vi "Generate volume table.vi"(8 "error in (no error)":errorcluster, 11 "Tomo in":refnum<class "Tomo.lvclass">) -> (0 "error out":errorcluster, 2 "Volume table":dbl[][](array[numeric]), 3 "Tomo out":refnum<class "Tomo.lvclass">)   [LabVIEW 2012, in "Tomo.lvclass"]
uses:
  Tomo.lvclass
  Tomo.lvclass/Tomo.ctl
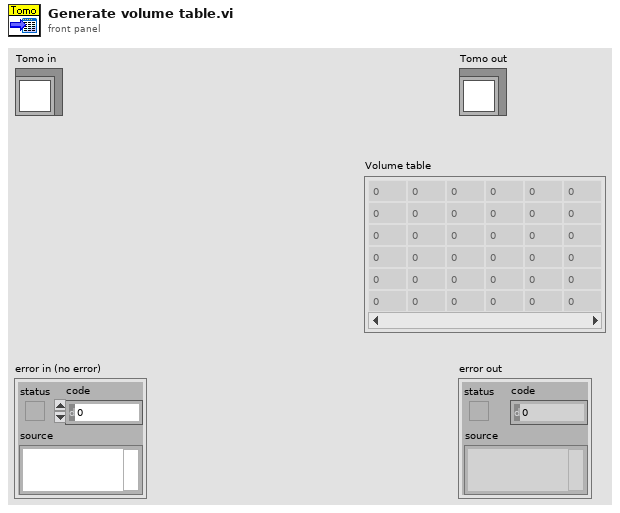
[diagram p1: front panel]
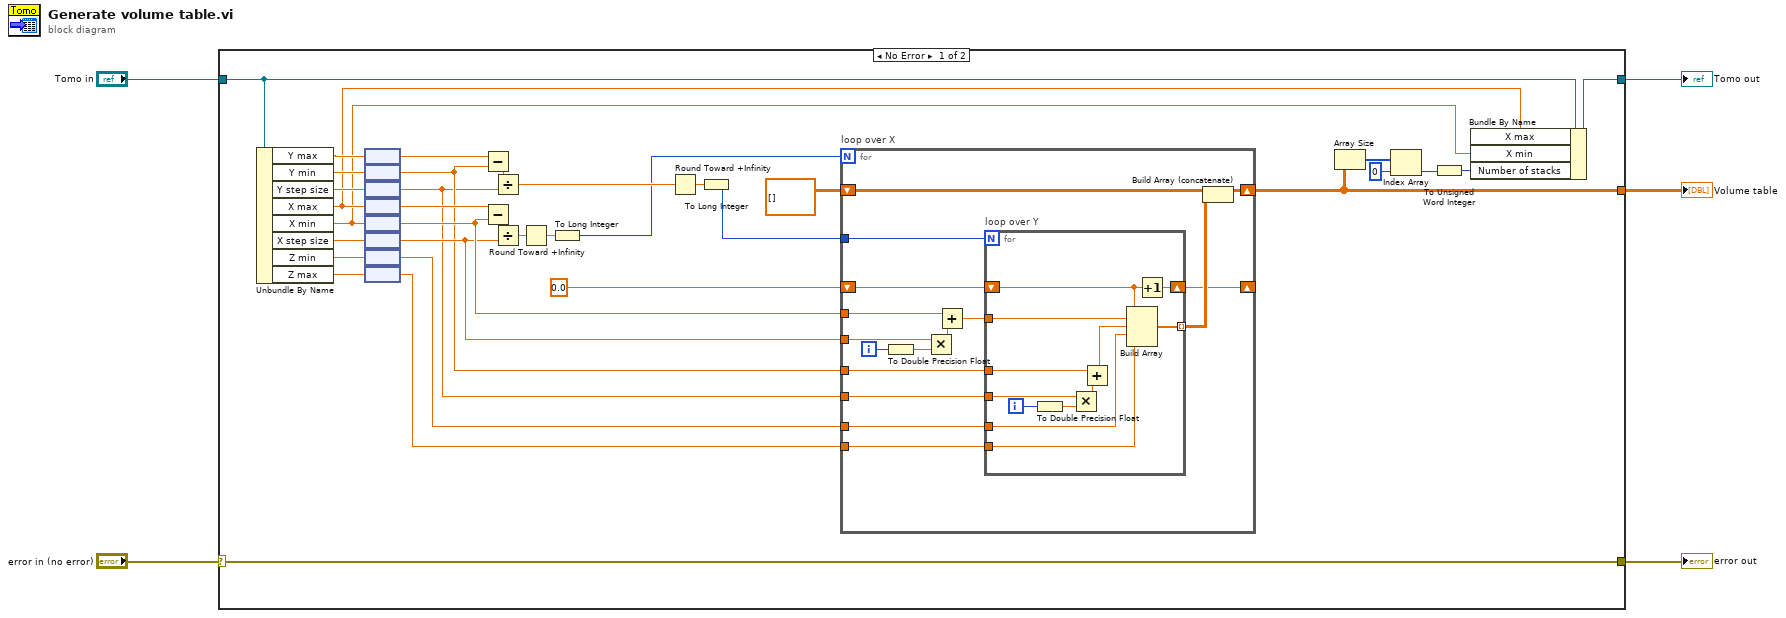
[diagram p0: block diagram]
diagram:
  n1 = case shown="No Error" "error in (no error)" {
    selector: "error in (no error)" -> [w39 w69]
    tunnel: [w39 w69] -> w4
    tunnel: [w12 w68] -> w2
    tunnel: "Tomo in" -> [w13 w68]
    tunnel: [w16 _] -> w1
    frame No Error {
      n2 = Unbundle By Name(w13) -> ("Y max"=w38:dbl[unit], "Y min"=w37:dbl[unit], "Y step size"=w36:dbl[unit], "X max"=w7:dbl[unit], "X min"=w6:dbl[unit], "X step size"=w27:dbl[unit], "Z min"=w21:dbl[unit], "Z max"=w19:dbl[unit])
      n3 = node(w38) -> (w28:dbl)
      n4 = node(w37) -> (w23:dbl)
      n5 = node(w36) -> (w22:dbl)
      n6 = node(w7) -> (w26:dbl)
      n7 = node(w6) -> (w25:dbl)
      n8 = node(w27) -> (w24:dbl)
      n9 = node(w21) -> (w20:dbl)
      n10 = node(w19) -> (w18:dbl)
      n11 = Subtract(x=w28, y=w23) -> (x-y=w35:dbl)
      n12 = Subtract(x=w26, y=w25) -> (x-y=w34:dbl)
      n13 = Divide(x=w35, y=w22) -> (x/y=w33:dbl)
      n14 = Divide(x=w34, y=w24) -> (x/y=w32:dbl)
      n15 = Round Toward +Infinity(x=w32) -> (ceil(x): smallest int >= x=w30:dbl)
      n16 = To Long Integer(number=w30) -> (32bit integer=w9:i32)
      n17 = Round Toward +Infinity(x=w33) -> (ceil(x): smallest int >= x=w31:dbl)
      n18 = To Long Integer(number=w31) -> (32bit integer=w8:i32)
      n19 = for "loop over X" {
        N: w9 -> [_]
        tunnel: w8 -> [w55]
        shift-right: [w40] -> _
        shift-left: 0.0 -> [w53]
        tunnel: w25 -> [w49]
        tunnel: w24 -> [w48]
        tunnel: w23 -> [w47]
        tunnel: w22 -> [w46]
        tunnel: w20 -> [w45]
        tunnel: w18 -> [w44]
        shift-right: [w43] -> w16
        shift-left: dbl[][] [] -> [w41]
        i -> [w54]
        n20 = To Double Precision Float(number=w54) -> (double precision float=w51:dbl)
        n21 = Multiply(x=w48, y=w51) -> (x*y=w52:dbl)
        n22 = Add(x=w49, y=w52) -> (x+y=w50:dbl)
        n23 = for "loop over Y" {
          N: w55 -> [_]
          shift-right: [w66] -> w40
          shift-left: w53 -> [w56]
          tunnel: w50 -> [w65]
          tunnel: w47 -> [w64]
          tunnel: w46 -> [w63]
          tunnel: w45 -> [w59]
          tunnel: w44 -> [w58]
          tunnel: [w57] -> w42 mode=indexing
          i -> [w67]
          n24 = To Double Precision Float(number=w67) -> (double precision float=w62:dbl)
          n25 = Multiply(x=w63, y=w62) -> (x*y=w61:dbl)
          n26 = Add(x=w64, y=w61) -> (x+y=w60:dbl)
          n27 = Build Array(w56, w65, w60, w59, w58) -> (w57:dbl[])
          n28 = Increment(x=w56) -> (x+1=w66:dbl)
        }
        n29 = Build Array (concatenate)(w41, w42) -> (w43:dbl[][])
      }
      n30 = Array Size(array=w16) -> (size(s)=w15:i32[])
      n31 = Index Array(array=w15, index=0) -> (element=w11:i32)
      n32 = To Unsigned Word Integer(number=w11) -> (unsigned 16bit integer=w10:u16)
      n33 = Bundle By Name(cluster=w13, "X max"=w7, "X min"=w6, "Number of stacks"=w10) -> (w12:refnum<class "Tomo.lvclass">)
    }
    frame Error {
    }
  }
  "error out" <- w4
  "Tomo out" <- w2
  "Volume table" <- w1
